vi "Test firmware upload.vi"(8 "error in":errorcluster) -> (0 "error out":errorcluster, 1 "Error Lin":i32, 2 "Pass?":bool, 3 ".128 file Path 2":path=path "E:/LCU6331 test/Procedure2/RFID_m645_Prodtest_LCU6331.128" caption="Path")   [LabVIEW 2009]
uses:
  Digit IO PCI 6503/Digit IO control.ctl
  Global/Global 1.vi
  <vilib>/Instr/_visa.llb/VISA Configure Serial Port (Instr).vi
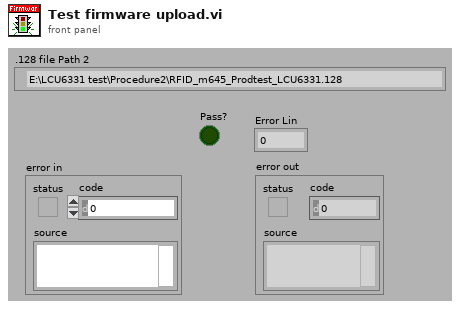
[diagram p1: front panel]
types:
  T1 = typedef "Digit IO control.ctl" = enum16{"Pull X1_4 Low", "Disconnect Pull X1_4 Low", "Down Cylinder", "Disconnect Down Cylinder", "Load X1_1_5", "Disconnect Load X1_1_5", "Measu X1_1_5", "Disconnect Measu X1_1_5", "Measu Z1_1_5", "Disconnect Measu Z1_1_5", "Power X1_1", "Disconnect Power X1_1", "RS232 Power", "Disconnect RS232 Power", "Card Cylinder", "Disconnect Card Cylinder", "Fail LED", "Disconnect Fail LED", "LCA Power", "Disconnect LCA Power", "BeyondCylinderDowndigit", "Disconnect BeyondCylinderDowendigit", "Frequency", "Disconnect Frequency", "Measu Current", "Disconnect Measu Current", "Measu current_1", "Disconnect Measu current_1", "Digit ALL", "Disconnect Digit ALL", "PASS LED", "Disconnect PASS LED", "Load Z1_1_3", "Disconnect Load Z1_1_3", "RS232 Connect", "Disconnect RS232 Connect", "Power Z1_7", "Disconnect Power Z1_7", "Pull Z_1_5  low", "Disconnect Pull Z_1_5  low", "Connect LCA_1", "Disconnect LCA_1", "short LCA", "Disconnect short LCA", "PT100", "Disconnect PT100", "NO connect", "Disconnect NO connect"}
  T2 = enum16{"Initialize", "Uploading 218 file", "Release X1.4", "Commnd_0 & Verify", "Finish"}
  T3 = cluster{".128 file":path, "Appliction firmware file":path, "Data file":path, "Txt path":path, "EXCEL path":path}
  T4 = cluster{"People":string, "product  number":string, "Test time":string, "VHeatFuse_noload":string, "VHeatFuse_load":string, "VoverrideDiode":string, "Test firmware upload via X1":string, "TemperAddress":string, "Troom":string, "TLCU":string, "Adjustment factor":string, "MeasuredFreq":string, "I2C communication":string, "Light-emitting diode on Z2":string, "Battery warning/inhibit":string, "Reset by IC10":string, "External EEPROM":string, "RFID card detection and reading RFID":string, "Production parameters in internal EEPROM":string, "Current consumption in sleep mode":string, "Application and database upload":string, "Test result":string, "Table head[22]":string, "Table head[23]":string}
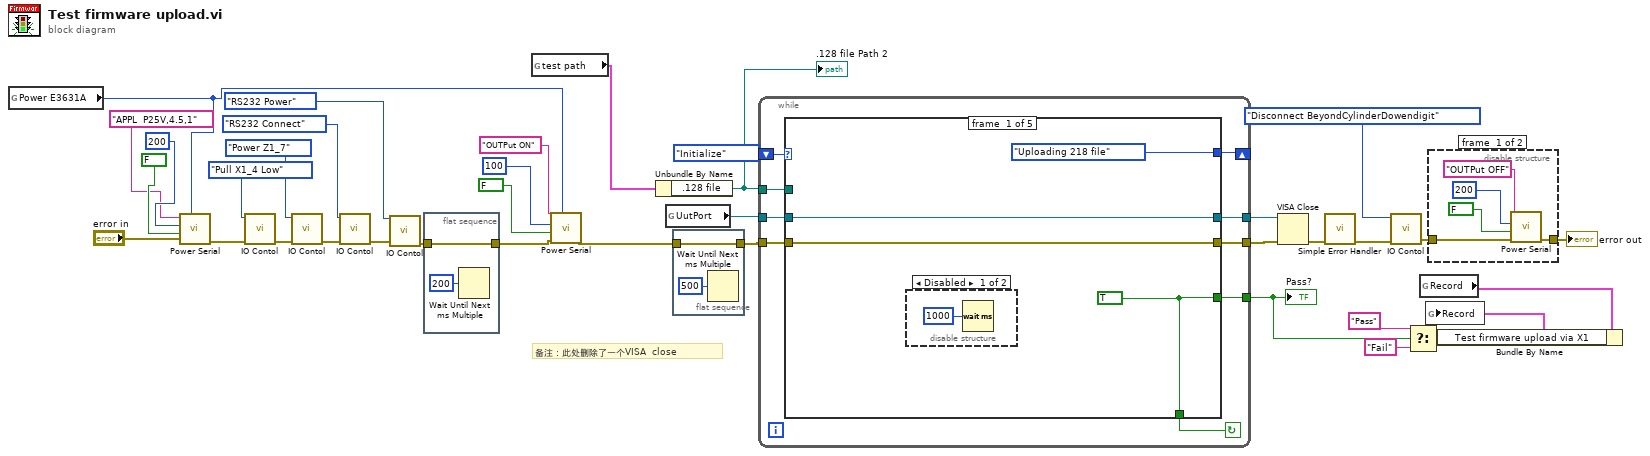
[diagram p0: block diagram]
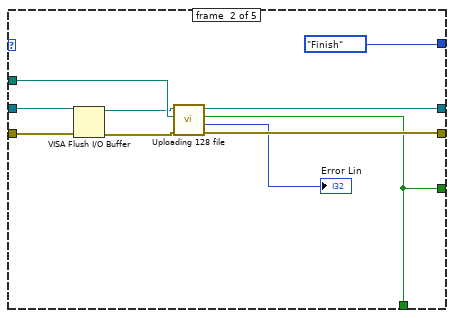
[diagram p4: hidden frame]
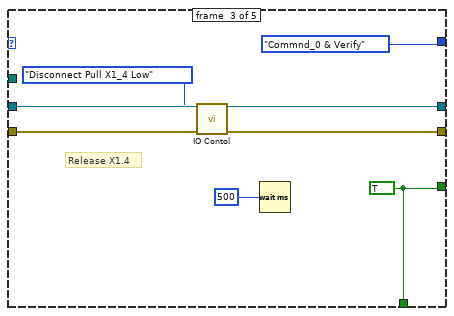
[diagram p5: hidden frame]
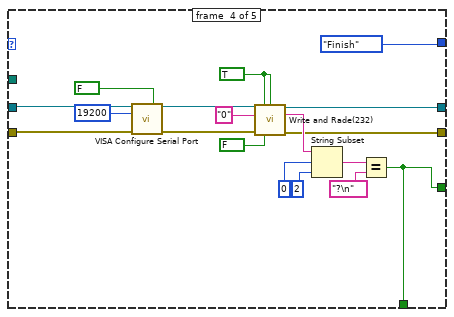
[diagram p6: hidden frame]
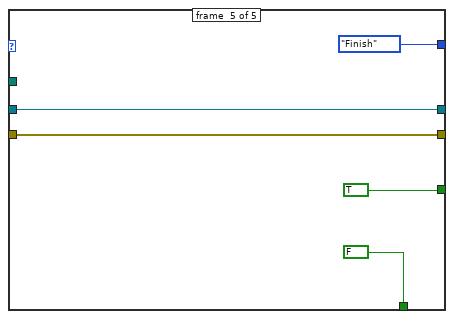
[diagram p7: hidden frame]
diagram:
  # "备注：此处删除了一个VISA  close"
  n1 = global read "Global 1.vi" "Power E3631A"() -> (w6:i32)
  n2 = call "Power Serial.vi"("VISA Resource Address"=w6, "error in (no error)"="error in", "Rd?"=FALSE, "Delay"=200, "IN"="APPL  P25V,4.5,1" ("In")) -> ("error out"=w26:errorcluster)  [unwired: 6 out]
  n3 = call "IO Contol.vi"("error in"=w26, "IO Operation"=Digit_IO_control."Pull X1_4 Low" ("Enum")) -> ("error out"=w20:errorcluster)  [unwired: 9 out]
  n4 = call "IO Contol.vi"("error in"=w20, "IO Operation"=Digit_IO_control."Power Z1_7" ("Enum")) -> ("error out"=w30:errorcluster)  [unwired: 9 out]
  n5 = call "IO Contol.vi"("error in"=w30, "IO Operation"=Digit_IO_control."RS232 Connect" ("Enum")) -> ("error out"=w25:errorcluster)  [unwired: 9 out]
  n6 = call "IO Contol.vi"("error in"=w25, "IO Operation"=Digit_IO_control."RS232 Power") -> ("error out"=w9:errorcluster)  [unwired: 9 out]
  n7 = flat-sequence {
    tunnel: w9 -> [w39]
    tunnel: [w39] -> w8
    frame #0 {
      n8 = Wait Until Next ms Multiple(millisecond multiple=u32 200) -> ()  [unwired: 1 out]
    }
  }
  n9 = global read "Global 1.vi" "test path"() -> (w3:T3)
  n10 = call "Power Serial.vi"("VISA Resource Address"=w6, "error in (no error)"=w8, "Rd?"=FALSE, "Delay"=100, "IN"="OUTPut ON" ("In")) -> ("error out"=w1:errorcluster)  [unwired: 6 out]
  n11 = Unbundle By Name(w3) -> (".128 file"=w2:path)
  ".128 file Path 2" <- w2
  n12 = global read "Global 1.vi" "UutPort"() -> (w7:refnum<visa-resource-name>)
  n13 = flat-sequence {
    tunnel: w1 -> [w41]
    tunnel: [w41] -> w5
    frame #0 {
      n14 = Wait Until Next ms Multiple(millisecond multiple=u32 500) -> ()  [unwired: 1 out]
    }
  }
  n15 = while {
    shift-right: [w42] -> _
    shift-left: T2."Initialize" -> [w50]
    tunnel: w7 -> [w48]
    tunnel: w5 -> [w47]
    tunnel: [w46] -> w35
    tunnel: [w45] -> w34
    tunnel: [w44] -> w15
    tunnel: w2 -> [w43]
    stop <- w49 continue-if-true
    n16 = case shown="\"Uploading 218 file\"" w50 {
      tunnel: [T2."Uploading 218 file" T2."Finish" T2."Commnd_0 & Verify" T2."Finish" T2."Finish"] -> w42
      tunnel: [w52 w62 w72 w81 FALSE] -> w49
      tunnel: w48 -> [w54 w59 w71 w77 w95]
      tunnel: w47 -> [w53 w57 w69 w76 w94]
      tunnel: [w54 w64 w71 w83 w95] -> w46
      tunnel: [w53 w63 w66 w82 w94] -> w45
      tunnel: [w52 w62 w72 w81 TRUE] -> w44
      tunnel: w43 -> [_ w65 _ _ _]
      frame #0 {
        w52 = TRUE
        n17 = disable-structure shown="Disabled" {
          frame #0 {
            n18 = Wait (ms)(milliseconds to wait=u32 1000) -> ()  [unwired: 1 out]
          }
          frame #1 {
          }
        }
      }
      frame #1 {
        n19 = VISA Flush I/O Buffer(VISA resource name=w59, error in (no error)=w57) -> (VISA resource name out=w58:refnum<visa-resource-name>, error out=w56:errorcluster)  [unwired: 1 out]
        n20 = call "Uploading 128 file.vi"("error in (no error)"=w56, ".128 file Path"=w65, "VISA resource name"=w58) -> ("error out"=w63:errorcluster, "Error Lin"=→"Error Lin":i32, "Pass?"=w62:bool, "VISA resource name out"=w64:refnum<visa-resource-name>)  [unwired: 5 out]
      }
      frame #2 {
        w72 = TRUE
        # "Release X1.4"
        n21 = call "IO Contol.vi"("error in"=w69, "IO Operation"=Digit_IO_control."Disconnect Pull X1_4 Low") -> ("error out"=w66:errorcluster)  [unwired: 9 out]
        n22 = Wait (ms)(milliseconds to wait=u32 500) -> ()  [unwired: 1 out]
      }
      frame #3 {
        w85 = TRUE ("write")
        n23 = call-poly "VISA Configure Serial Port"("VISA resource name"=w77, "Enable Termination\nChar (T)"=FALSE ("Enable Termination\nChar (T)"), "baud rate (9600)"=u32 19200, "error in (no error)"=w76) -> ("VISA resource name out"=w75:refnum<visa-resource-name>, "error out"=w74:errorcluster)  [unwired: 3 in, 7 out]
        n24 = call "Write and Rade(232).vi"("VISA resource name in"=w75, "write"=w85, "read"=w85, "string to write"="0", "error in"=w74, "change baud rate(read)"=FALSE) -> ("VISA resource name out"=w83:refnum<visa-resource-name>, "read string"=w86:string, "error out"=w82:errorcluster)  [unwired: 2 in, 5 out]
        n25 = String Subset(string=w86, offset (0)=0, length (rest)=2 ("length (rest)")) -> (substring=w88:string)
        n26 = Equal?(x=w88, y="?\n") -> (x = y?=w81:bool)
      }
      frame #4 {
      }
    }
  }
  "Pass?" <- w15
  n27 = VISA Close(VISA resource name=w35, error in (no error)=w34) -> (error out=w36:errorcluster)
  n28 = call <vilib>:"Simple Error Handler.vi"("error in (no error)"=w36) -> ("error out"=w18:errorcluster)  [unwired: 1 in, 7 out]
  n29 = call "IO Contol.vi"("error in"=w18, "IO Operation"=Digit_IO_control."Disconnect BeyondCylinderDowendigit") -> ("error out"=w19:errorcluster)  [unwired: 9 out]
  n30 = Select(t="Pass", s=w15, f="Fail") -> (s? t:f=w11:string)
  n31 = global read "Global 1.vi" "Record"() -> (w12:T4)
  n32 = disable-structure shown="Enabled" {
    disable-tunnel: w19 -> [w97 w101]
    disable-tunnel: [w96 w101] -> w17
    frame #0 {
      n33 = call "Power Serial.vi"("error in (no error)"=w97, "Rd?"=FALSE, "Delay"=200, "IN"="OUTPut OFF" ("In")) -> ("error out"=w96:errorcluster)  [unwired: 6 in, 1 out]
    }
    frame #1 {
    }
  }
  "error out" <- w17
  n34 = Bundle By Name(cluster=w12, "Test firmware upload via X1"=w11) -> (w10:T4)
  n35 = global write "Global 1.vi" "Record"(w10) -> ()
